vi "Next.vi"(8 "error in (no error)":errorcluster, 11 "LUnit Test Case In":refnum<class "LUnit Test Case.lvclass">) -> (0 "error out":errorcluster, 1 "Suite":string, 2 "Name":string, 3 "LUnit Test Case Out":refnum<class "LUnit Test Case.lvclass">)   [LabVIEW 2020, in "LUnit Test Case.lvclass"]
uses:
  LUnit Test Case.lvclass
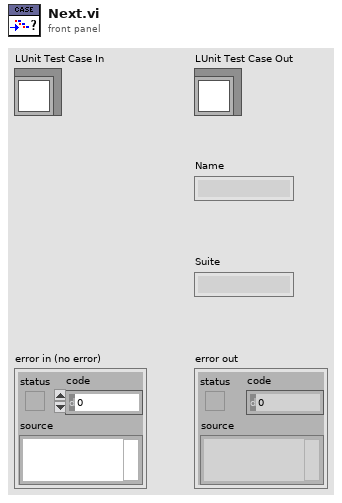
[diagram p1: front panel]
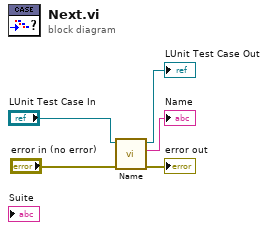
[diagram p0: block diagram]
diagram:
  n1 = call-dynamic "Name.vi"("error in (no error)"="error in (no error)", "LUnit Test Case in"="LUnit Test Case In") -> ("error out"=→"error out":errorcluster, "Name"=→"Name":string, "LUnit Test Case out"=→"LUnit Test Case Out":refnum<class "LUnit Test Case.lvclass">)  [unwired: 7 in]
